vi "Error_mx.vi"() -> ()   [LabVIEW 2021]
uses:
  <vilib>/Utility/miscctls.llb/LVDateTimeRec.ctl
panel:
  out "Elapsed Time (s)":dbl caption="已用时间(s)"
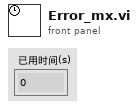
[diagram p1: front panel]
types:
  T1 = typedef "LVDateTimeRec.ctl" = cluster{"fractional second":dbl, "second":i32, "minute":i32, "hour":i32, "day of month":i32, "month":i32, "year":i32, "day of week":i32, "day of year":i32, "DST":i32}
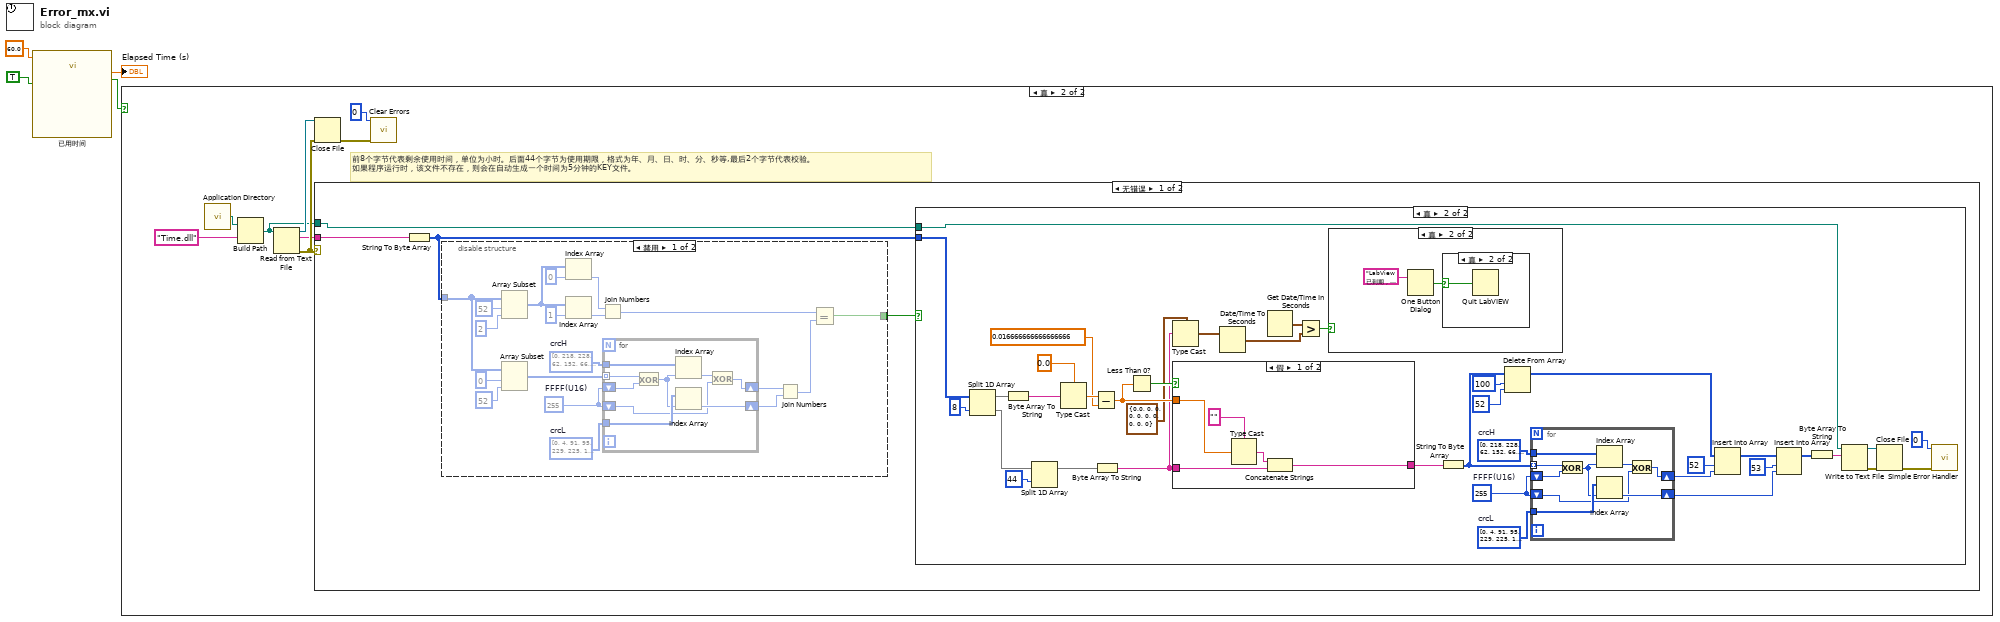
[diagram p0: block diagram]
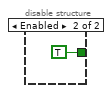
[diagram p3: hidden frame]
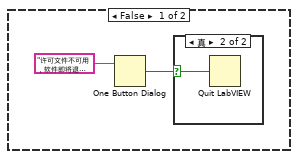
[diagram p4: hidden frame]
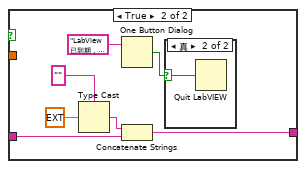
[diagram p8: hidden frame]
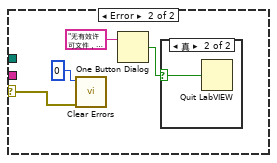
[diagram p10: hidden frame]
diagram:
  n1 = call "已用时间"("Time Target (s)"=60.0, "Auto Reset"=TRUE) -> ("Elapsed Time (s)"=→"Elapsed Time (s)":dbl, "Time has Elapsed"=w1:bool)  [unwired: 10 in, 6 out]
  n2 = case shown="真" w1 {
    frame False {
    }
    frame True {
      # "前8个字节代表剩余使用时间，单位为小时。后面44个字节为使用期限，格式为年、月、日、时、分、秒等,最后2个字节代表校验。\n如果程序运行时，该文件不存在，则会在自动生成一个时间为5分钟的KEY文件。"
      n3 = call <vilib>:"Application Directory.vi"() -> ("Application Directory"=w12:path)
      n4 = Build Path(base path=w12, name or relative path="Time.dll" ("名称或相对路径")) -> (appended path=w5:path)
      n5 = Read from Text File(file (use dialog)=w5) -> (refnum out=w9:refnum<file>, text=w6:string, error out=w10:errorcluster)  [unwired: 3 in, 1 out]
      n6 = Close File(refnum=w9, error in=w10) -> (error out=w8:errorcluster)  [unwired: 1 out]
      n7 = case shown="无错误" w10 {
        selector: w10 -> [_ w115]
        tunnel: w6 -> [w16 _]
        tunnel: w5 -> [w15 _]
        frame No Error {
          n8 = String To Byte Array(string=w16) -> (unsigned byte array=w14:u8[])
          n9 = disable-structure shown="禁用" {
            disable-tunnel: w14 -> [w29 _]
            disable-tunnel: [w17 TRUE] -> w13
            frame Disabled {
              w32 = u8[] [0, 4, 91, 95, 229, 225, 190, 186, 153, 157, 194, 198, 124, 120, 39, 35, 50, 54, 105, 109, 215, 211, 140, 136, 171, 175, 240, 244, 78, 74, 21, 17, 55, 51, 108, 104, 210, 214, 137, 141, 174, 170, 245, 241, 75, 79, 16, 20, 5, 1, 94, 90, 224, 228, 187, 191, 156, 152, 199, 195, 121, 125, 34, 38, 61, 57, 102, 98, 216, 220, 131, 135, 164, 160, 255, 251, 65, 69, 26, 30, 15, 11, 84, 80, 234, 238, 177, 181, 150, 146, 205, 201, 115, 119, 40, 44, 10, 14, 81, 85, 239, 235, 180, 176, 147, 151, 200, 204, 118, 114, 45, 41, 56, 60, 99, 103, 221, 217, 134, 130, 161, 165, 250, 254, 68, 64, 31, 27, 41, 45, 114, 118, 204, 200, 151, 147, 176, 180, 235, 239, 85, 81, 14, 10, 27, 31, 64, 68, 254, 250, 165, 161, 130, 134, 217, 221, 103, 99, 60, 56, 30, 26, 69, 65, 251, 255, 160, 164, 135, 131, 220, 216, 98, 102, 57, 61, 44, 40, 119, 115, 201, 205, 146, 150, 181, 177, 238, 234, 80, 84, 11, 15, 20, 16, 79, 75, 241, 245, 170, 174, 141, 137, 214, 210, 104, 108, 51, 55, 38, 34, 125, 121, 195, 199, 152, 156, 191, 187, 228, 224, 90, 94, 1, 5, 35, 39, 120, 124, 198, 194, 157, 153, 186, 190, 225, 229, 95, 91, 4, 0, 17, 21, 74, 78, 244, 240, 175, 171, 136, 140, 211, 215, 109, 105, 54, 50]  # crcL
              w33 = u8[] [0, 218, 228, 62, 152, 66, 124, 166, 97, 187, 133, 95, 249, 35, 29, 199, 195, 25, 39, 253, 91, 129, 191, 101, 162, 120, 70, 156, 58, 224, 222, 4, 214, 12, 50, 232, 78, 148, 170, 112, 183, 109, 83, 137, 47, 245, 203, 17, 21, 207, 241, 43, 141, 87, 105, 179, 116, 174, 144, 74, 236, 54, 8, 210, 252, 38, 24, 194, 100, 190, 128, 90, 157, 71, 121, 163, 5, 223, 225, 59, 63, 229, 219, 1, 167, 125, 67, 153, 94, 132, 186, 96, 198, 28, 34, 248, 42, 240, 206, 20, 178, 104, 86, 140, 75, 145, 175, 117, 211, 9, 55, 237, 233, 51, 13, 215, 113, 171, 149, 79, 136, 82, 108, 182, 16, 202, 244, 46, 168, 114, 76, 150, 48, 234, 212, 14, 201, 19, 45, 247, 81, 139, 181, 111, 107, 177, 143, 85, 243, 41, 23, 205, 10, 208, 238, 52, 146, 72, 118, 172, 126, 164, 154, 64, 230, 60, 2, 216, 31, 197, 251, 33, 135, 93, 99, 185, 189, 103, 89, 131, 37, 255, 193, 27, 220, 6, 56, 226, 68, 158, 160, 122, 84, 142, 176, 106, 204, 22, 40, 242, 53, 239, 209, 11, 173, 119, 73, 147, 151, 77, 115, 169, 15, 213, 235, 49, 246, 44, 18, 200, 110, 180, 138, 80, 130, 88, 102, 188, 26, 192, 254, 36, 227, 57, 7, 221, 123, 161, 159, 69, 65, 155, 165, 127, 217, 3, 61, 231, 32, 250, 196, 30, 184, 98, 92, 134]  # crcH
              w31 = u8 255  # FFFF(U16)
              n10 = Array Subset(array=w29, index=52 ("索引"), length=2 ("长度")) -> (w24:u8[])
              n11 = Array Subset(array=w29, index=0 ("索引"), length=52 ("长度")) -> (w30:u8[])
              n12 = Index Array(array=w24, index=0 ("索引")) -> (element=w23:u8)
              n13 = Index Array(array=w24, index=1 ("索引")) -> (element=w22:u8)
              n14 = Join Numbers(hi=w23, lo=w22) -> ((hi.lo)=w21:u16)
              n15 = for {
                tunnel: w30 -> [w43] mode=indexing
                tunnel: w33 -> [w42]
                tunnel: w32 -> [w41]
                shift-right: [w37] -> w20
                shift-left: w31 -> [w36]
                shift-right: [w38] -> w19
                shift-left: w31 -> [w44]
                n16 = Exclusive Or(1:w44, 2:w43) -> (0:w40:u8)
                n17 = Index Array(array=w42, index=w40) -> (element=w39:u8)
                n18 = Index Array(array=w41, index=w40) -> (element=w37:u8)
                n19 = Exclusive Or(1:w36, 2:w39) -> (0:w38:u8)
              }
              n20 = Join Numbers(hi=w19, lo=w20) -> ((hi.lo)=w18:u16)
              n21 = Equal?(x=w21, y=w18) -> (x = y?=w17:bool)
            }
            frame Enabled {
            }
          }
          n22 = case shown="真" w13 {
            tunnel: w15 -> [_ w71]
            tunnel: w14 -> [_ w67]
            frame False {
              n23 = One Button Dialog(message="许可文件不可用，软件即将退出。" ("消息")) -> (true=w46:bool)  [unwired: 1 in]
              n24 = case shown="真" w46 {
                selector: w46 -> [_ w48]
                frame False {
                }
                frame True {
                  n25 = Quit LabVIEW(quit? (T)=w48) -> ()
                }
              }
            }
            frame True {
              w60 = u8[] [0, 4, 91, 95, 229, 225, 190, 186, 153, 157, 194, 198, 124, 120, 39, 35, 50, 54, 105, 109, 215, 211, 140, 136, 171, 175, 240, 244, 78, 74, 21, 17, 55, 51, 108, 104, 210, 214, 137, 141, 174, 170, 245, 241, 75, 79, 16, 20, 5, 1, 94, 90, 224, 228, 187, 191, 156, 152, 199, 195, 121, 125, 34, 38, 61, 57, 102, 98, 216, 220, 131, 135, 164, 160, 255, 251, 65, 69, 26, 30, 15, 11, 84, 80, 234, 238, 177, 181, 150, 146, 205, 201, 115, 119, 40, 44, 10, 14, 81, 85, 239, 235, 180, 176, 147, 151, 200, 204, 118, 114, 45, 41, 56, 60, 99, 103, 221, 217, 134, 130, 161, 165, 250, 254, 68, 64, 31, 27, 41, 45, 114, 118, 204, 200, 151, 147, 176, 180, 235, 239, 85, 81, 14, 10, 27, 31, 64, 68, 254, 250, 165, 161, 130, 134, 217, 221, 103, 99, 60, 56, 30, 26, 69, 65, 251, 255, 160, 164, 135, 131, 220, 216, 98, 102, 57, 61, 44, 40, 119, 115, 201, 205, 146, 150, 181, 177, 238, 234, 80, 84, 11, 15, 20, 16, 79, 75, 241, 245, 170, 174, 141, 137, 214, 210, 104, 108, 51, 55, 38, 34, 125, 121, 195, 199, 152, 156, 191, 187, 228, 224, 90, 94, 1, 5, 35, 39, 120, 124, 198, 194, 157, 153, 186, 190, 225, 229, 95, 91, 4, 0, 17, 21, 74, 78, 244, 240, 175, 171, 136, 140, 211, 215, 109, 105, 54, 50]  # crcL
              w61 = u8[] [0, 218, 228, 62, 152, 66, 124, 166, 97, 187, 133, 95, 249, 35, 29, 199, 195, 25, 39, 253, 91, 129, 191, 101, 162, 120, 70, 156, 58, 224, 222, 4, 214, 12, 50, 232, 78, 148, 170, 112, 183, 109, 83, 137, 47, 245, 203, 17, 21, 207, 241, 43, 141, 87, 105, 179, 116, 174, 144, 74, 236, 54, 8, 210, 252, 38, 24, 194, 100, 190, 128, 90, 157, 71, 121, 163, 5, 223, 225, 59, 63, 229, 219, 1, 167, 125, 67, 153, 94, 132, 186, 96, 198, 28, 34, 248, 42, 240, 206, 20, 178, 104, 86, 140, 75, 145, 175, 117, 211, 9, 55, 237, 233, 51, 13, 215, 113, 171, 149, 79, 136, 82, 108, 182, 16, 202, 244, 46, 168, 114, 76, 150, 48, 234, 212, 14, 201, 19, 45, 247, 81, 139, 181, 111, 107, 177, 143, 85, 243, 41, 23, 205, 10, 208, 238, 52, 146, 72, 118, 172, 126, 164, 154, 64, 230, 60, 2, 216, 31, 197, 251, 33, 135, 93, 99, 185, 189, 103, 89, 131, 37, 255, 193, 27, 220, 6, 56, 226, 68, 158, 160, 122, 84, 142, 176, 106, 204, 22, 40, 242, 53, 239, 209, 11, 173, 119, 73, 147, 151, 77, 115, 169, 15, 213, 235, 49, 246, 44, 18, 200, 110, 180, 138, 80, 130, 88, 102, 188, 26, 192, 254, 36, 227, 57, 7, 221, 123, 161, 159, 69, 65, 155, 165, 127, 217, 3, 61, 231, 32, 250, 196, 30, 184, 98, 92, 134]  # crcH
              w59 = u8 255  # FFFF(U16)
              n26 = Split 1D Array(array=w67, index=8 ("索引")) -> (first subarray=w85:u8[], second subarray=w64:u8[])
              n27 = Byte Array To String(unsigned byte array=w85) -> (string=w73:string)
              n28 = Split 1D Array(array=w64, index=44 ("索引")) -> (first subarray=w62:u8[])  [unwired: 1 out]
              n29 = Type Cast(type=0.0, x=w73) -> (*(type *) &x=w83:dbl)
              n30 = Subtract(x=w83, y=0.016666666666666666) -> (x-y=w79:dbl)
              n31 = Byte Array To String(unsigned byte array=w62) -> (string=w72:string)
              n32 = Less Than 0?(x=w79) -> (x < 0?=w78:bool)
              n33 = Type Cast(type=T1 {"fractional second"=0.0, "second"=0, "minute"=0, "hour"=0, "day of month"=0, "month"=0, "year"=0, "day of week"=0, "day of year"=0, "DST"=0} ("日期时间记录"), x=w72) -> (*(type *) &x=w84:T1)
              n34 = case shown="假" w78 {
                tunnel: w79 -> [w102 _]
                tunnel: [w99 w106] -> w66
                tunnel: w72 -> [w100 w107]
                frame False {
                  n35 = Type Cast(type="", x=w102) -> (*(type *) &x=w101:string)
                  n36 = Concatenate Strings(w101, w100) -> (w99:string)
                }
                frame True {
                  n37 = Type Cast(type="", x=ext 0.0) -> (*(type *) &x=w108:string)
                  n38 = One Button Dialog(message="LabView已到期，请使用正版软件！" ("消息")) -> (true=w104:bool)  [unwired: 1 in]
                  n39 = Concatenate Strings(w108, w107) -> (w106:string)
                  n40 = case shown="真" w104 {
                    selector: w104 -> [_ w111]
                    frame False {
                    }
                    frame True {
                      n41 = Quit LabVIEW(quit? (T)=w111) -> ()
                    }
                  }
                }
              }
              n42 = Date/Time To Seconds(2:w84) -> (0:w70:timestamp)  [unwired: 1 in]
              n43 = Get Date/Time In Seconds() -> (seconds since 1Jan1904=w69:timestamp)
              n44 = Greater?(x=w69, y=w70) -> (0:w68:bool)
              n45 = case shown="真" w68 {
                frame False {
                }
                frame True {
                  n46 = One Button Dialog(message="LabView已到期，请使用正版软件！" ("消息")) -> (true=w96:bool)  [unwired: 1 in]
                  n47 = case shown="真" w96 {
                    selector: w96 -> [_ w98]
                    frame False {
                    }
                    frame True {
                      n48 = Quit LabVIEW(quit? (T)=w98) -> ()
                    }
                  }
                }
              }
              n49 = String To Byte Array(string=w66) -> (unsigned byte array=w52:u8[])
              n50 = Delete From Array(array=w52, length=100 ("长度"), index=52 ("索引")) -> (array with subset deleted=w50:u8[])  [unwired: 1 out]
              n51 = for {
                tunnel: w52 -> [w94] mode=indexing
                tunnel: w61 -> [w93]
                tunnel: w60 -> [w92]
                shift-right: [w88] -> w53
                shift-left: w59 -> [w87]
                shift-right: [w89] -> w54
                shift-left: w59 -> [w95]
                n52 = Exclusive Or(1:w95, 2:w94) -> (0:w91:u8)
                n53 = Index Array(array=w93, index=w91) -> (element=w90:u8)
                n54 = Index Array(array=w92, index=w91) -> (element=w88:u8)
                n55 = Exclusive Or(1:w87, 2:w90) -> (0:w89:u8)
              }
              n56 = Insert Into Array(array=w50, index=52 ("索引"), new element=w54) -> (w56:u8[])
              n57 = Insert Into Array(array=w56, index=53 ("索引"), new element=w53) -> (w55:u8[])
              n58 = Byte Array To String(unsigned byte array=w55) -> (string=w65:string)
              n59 = Write to Text File(file (use dialog)=w71, text=w65) -> (refnum out=w80:refnum<file>, error out=w81:errorcluster)  [unwired: 2 in, 1 out]
              n60 = Close File(refnum=w80, error in=w81) -> (error out=w82:errorcluster)  [unwired: 1 out]
              n61 = call <vilib>:"Simple Error Handler.vi"("error code (no error:0)"=0, "error in (no error)"=w82) -> ()  [unwired: 3 in, 5 out]
            }
          }
        }
        frame Error {
          n62 = call <vilib>:"Clear Errors.vi"("error in (no error)"=w115, "specific error code to clear (0: all)"=0) -> ()  [unwired: 4 in, 2 out]
          n63 = One Button Dialog(message="无有效许可文件，软件即将退出。" ("消息")) -> (true=w112:bool)  [unwired: 1 in]
          n64 = case shown="真" w112 {
            selector: w112 -> [_ w116]
            frame False {
            }
            frame True {
              n65 = Quit LabVIEW(quit? (T)=w116) -> ()
            }
          }
        }
      }
      n66 = call <vilib>:"Clear Errors.vi"("error in (no error)"=w8, "specific error code to clear (0: all)"=0) -> ()  [unwired: 4 in, 2 out]
    }
  }
